vi "Talker.vi"(0 "Add in":refnum<class "Add.lvclass">, 5 "Subpanel Ref":refnum<vi>, 11 "Error In":errorcluster) -> (4 "Add out":refnum<class "Add.lvclass">, 15 "Error Out":errorcluster)   [LabVIEW 2020, in "Add.lvclass"]
doc: "Method to call the UI Method. This will pass the object to the UI Method which will do the operation and return the object to the main vi."
uses:
  Add.lvclass
  UI.vi
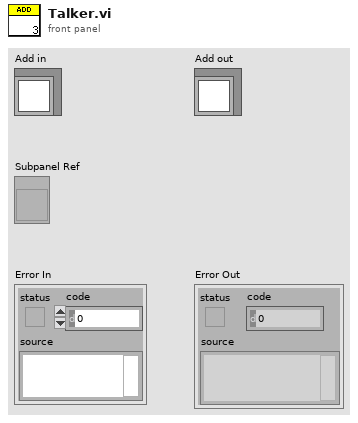
[diagram p1: front panel]
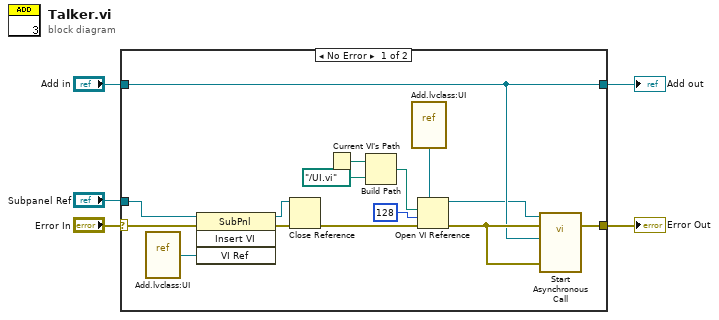
[diagram p0: block diagram]
diagram:
  n1 = case shown="No Error" "Error In" {
    selector: "Error In" -> [w16 w22]
    tunnel: [w19 w22] -> w4
    tunnel: [w18 w21] -> w2
    tunnel: "Add in" -> [w18 w21]
    tunnel: "Subpanel Ref" -> [w14 _]
    frame No Error {
      n2 = vi-ref "Add.lvclass:UI.vi"() -> (w6:refnum<vi>)
      n3 = invoke on="Invoke Node" class="SubPnl" method="Insert VI"(reference=w14, error in=w16, "VI Ref"=w6) -> (reference out=w10:refnum<vi>, error out=w15:errorcluster)  [unwired: 1 in, 2 out]
      n4 = Close Reference(reference=w10, error in (no error)=w15) -> (error out=w11:errorcluster)
      n5 = Current VI's Path() -> (path=w8:path)
      n6 = Build Path(base path=w8, name or relative path=path "../UI.vi") -> (appended path=w12:path)
      n7 = vi-ref "Add.lvclass:UI.vi"() -> (w9:refnum<vi>)
      n8 = Open VI Reference(type specifier VI Refnum (for type only)=w9, vi path=w12, options=128, error in (no error)=w11) -> (vi reference=w13:refnum<vi>, error out=w20:errorcluster)  [unwired: 2 in]
      n9 = call-by-ref "Start Asynchronous Call"(reference=w13, error in=w20, "Add.lvclass"=w18, "Error In"=w20) -> (error out=w19:errorcluster)  [unwired: 11 in, 4 out]
    }
    frame Error {
    }
  }
  "Error Out" <- w4
  "Add out" <- w2
